vi "CRYSearch for Intersection of Wave.vi"(4 "All points":bool, 6 "Search range":string[](array[string]), 7 "Supress warnings (F)":bool, 9 "Waveform B":T1={"Waveform"={"X0"=0.0, "dX"=0.0, "Y"=[]}, "X data"=1, "Y data"=0, "Y axis"=0, "X unit"="s", "Y unit"="", "Y dB ref"=1.0, "display Y"=TRUE, "display X"=FALSE, "Overload?"=FALSE, "Test Info"="", "Step No."=0, "Name"="", "protected"=FALSE, "Sqc history"=[], "Signal Channel ID"=0, "Plot Settings"={"Color"=0, "Interpolation"=0, "Point Style"=0, "Line Style"=0, "Point Color"=0, "Line Width"=0, "Bar Plot Style"=0, "Fill To"=0}, "AutoProtect"=FALSE} {"Y dB ref" format="%.1f"; "Y axis" items=["Log", "Lin"]; "Y data" items=["dB", "Lin"]; "X data" items=["dB", "Lin"]}, 11 "Waveform A":T1={"Waveform"={"X0"=0.0, "dX"=0.0, "Y"=[]}, "X data"=1, "Y data"=0, "Y axis"=0, "X unit"="s", "Y unit"="", "Y dB ref"=1.0, "display Y"=TRUE, "display X"=FALSE, "Overload?"=FALSE, "Test Info"="", "Step No."=0, "Name"="", "protected"=FALSE, "Sqc history"=[], "Signal Channel ID"=0, "Plot Settings"={"Color"=0, "Interpolation"=0, "Point Style"=0, "Line Style"=0, "Point Color"=0, "Line Width"=0, "Bar Plot Style"=0, "Fill To"=0}, "AutoProtect"=FALSE} {"Y dB ref" format="%.1f"; "Y axis" items=["Log", "Lin"]; "Y data" items=["dB", "Lin"]; "X data" items=["dB", "Lin"]}) -> (3 "Resulting data":T2={"Name"="", "Curve"=[], "X data"=1, "Y data"=1, "Z data"=1, "X axis"=0, "Y axis"=1, "Z axis"=1, "X unit"="Hz", "Y unit"="", "Z unit"="deg.", "X dB ref"=1.0, "Y dB ref"=1.0, "Z dB ref"=1.0, "single val"=FALSE, "protected"=FALSE, "display X"=TRUE, "display Y"=TRUE, "display Z"=TRUE, "Test Info"="", "Step No."=0, "Plot Settings"={"Color"=0, "Interpolation"=0, "Point Style"=0, "Line Style"=0, "Point Color"=0, "Line Width"=0, "Bar Plot Style"=0, "Fill To"=0}, "AutoProtect"=FALSE} {"Z data" items=["dB", "Lin"]; "X data" items=["dB", "Lin"]; "Y data" items=["dB", "Lin"]; "Z dB ref" format="%.1f"; "Z axis" items=["Log", "Lin"]; "X dB ref" format="%.1f"; "X axis" items=["Log", "Lin"]; "Y axis" items=["Log", "Lin"]; "Y dB ref" format="%.1f"; "Curve"."z" format="%.2f"; "Curve"."y" format="%.2f"; "Curve"."x" format="%.2f"})   [LabVIEW 2013]
uses:
  Typedef Control/CRYData Cluster.ctl
  Typedef Control/CRYWaveform Cluster.ctl
  <vilib>/Analysis/7linalg.llb/Solve Linear Equations (single right hand).vi
  <vilib>/Analysis/baseanly.llb/Solve Linear Equations By Cholesky.vi
  <vilib>/Analysis/baseanly.llb/Real Matrix to Compact Array.vi
  <vilib>/Analysis/baseanly.llb/Real Compact Tri-Matrix Linear Eqs.vi
  <vilib>/Analysis/7linalg.llb/Solve Linear Eqs (General).vi
  <vilib>/Analysis/7linalg.llb/Solve Linear Eqs (Gen, single right hand).vi
  <vilib>/Analysis/NI_AALPro.lvlib
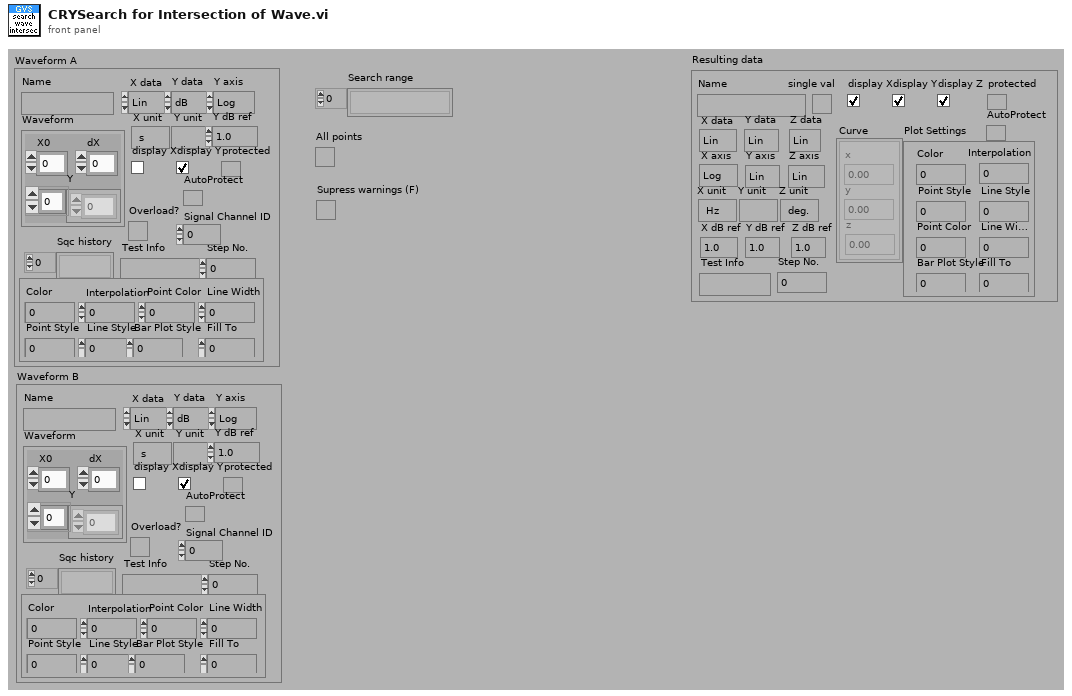
[diagram p1: front panel]
types:
  T1 = typedef "CRYWaveform Cluster.ctl" = cluster{"Waveform":cluster{"X0":dbl, "dX":dbl, "Y":sgl[]}, "X data":u16, "Y data":u16, "Y axis":u16, "X unit":string, "Y unit":string, "Y dB ref":dbl, "display Y":bool, "display X":bool, "Overload?":bool, "Test Info":string, "Step No.":i32, "Name":string, "protected":bool, "Sqc history":string[], "Signal Channel ID":i32, "Plot Settings":cluster{"Color":u32, "Interpolation":u8, "Point Style":u8, "Line Style":u8, "Point Color":u32, "Line Width":u8, "Bar Plot Style":u8, "Fill To":i16}, "AutoProtect":bool}
  T2 = typedef "CRYData Cluster.ctl" = cluster{"Name":string, "Curve":cluster{"x":dbl, "y":dbl, "z":dbl}[], "X data":u16, "Y data":u16, "Z data":u16, "X axis":u16, "Y axis":u16, "Z axis":u16, "X unit":string, "Y unit":string, "Z unit":string, "X dB ref":dbl, "Y dB ref":dbl, "Z dB ref":dbl, "single val":bool, "protected":bool, "display X":bool, "display Y":bool, "display Z":bool, "Test Info":string, "Step No.":i32, "Plot Settings":cluster{"Color":u32, "Interpolation":u8, "Point Style":u8, "Line Style":u8, "Point Color":u32, "Line Width":u8, "Bar Plot Style":u8, "Fill To":i16}, "AutoProtect":bool}
  T3 = enum16{"OK", "Yes", "YesNo", "YesNoCancel", "ReplaceAppend"}
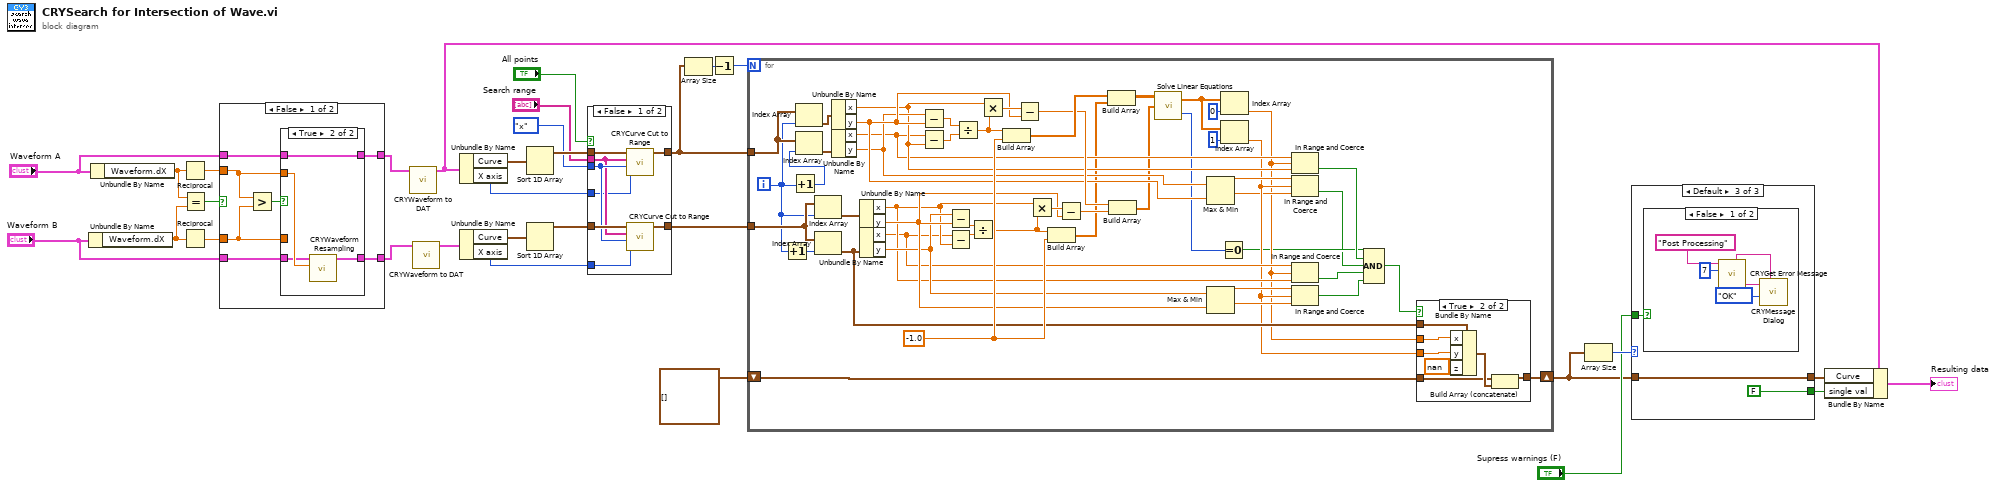
[diagram p0: block diagram]
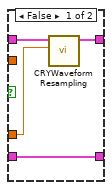
[diagram p3: hidden frame]
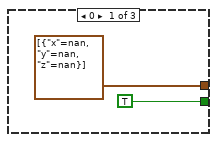
[diagram p5: hidden frame]
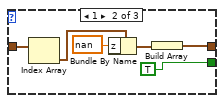
[diagram p6: hidden frame]
diagram:
  n1 = Unbundle By Name("Waveform B") -> ("Waveform.dX"=w13:dbl)
  n2 = Unbundle By Name("Waveform A") -> ("Waveform.dX"=w14:dbl)
  n3 = Reciprocal(x=w14) -> (1/x=w12:dbl)
  n4 = Reciprocal(x=w13) -> (1/x=w11:dbl)
  n5 = Equal?(x=w14, y=w13) -> (x = y?=w1:bool)
  n6 = case shown="False" w1 {
    tunnel: "Waveform A" -> [w38 w48]
    tunnel: "Waveform B" -> [w35 w47]
    tunnel: [w37 w48] -> w10
    tunnel: [w34 w47] -> w9
    tunnel: w12 -> [w36 _]
    tunnel: w11 -> [w33 _]
    frame False {
      n7 = Greater?(x=w36, y=w33) -> (0:w32:bool)
      n8 = case shown="True" w32 {
        tunnel: w38 -> [w42 w46]
        tunnel: [w40 w46] -> w37
        tunnel: w36 -> [_ w45]
        tunnel: w35 -> [w39 w44]
        tunnel: [w39 w43] -> w34
        tunnel: w33 -> [w41 _]
        frame False {
          n9 = call "CRYWaveform Resampling.vi"("New Sampling Rate"=w41, "Wave"=w42) -> ("New Wave"=w40:T1)  [unwired: 9 in]
        }
        frame True {
          n10 = call "CRYWaveform Resampling.vi"("New Sampling Rate"=w45, "Wave"=w44) -> ("New Wave"=w43:T1)  [unwired: 9 in]
        }
      }
    }
    frame True {
    }
  }
  n11 = call "CRYWaveform to DAT.vi"("Waveform In"=w10) -> ("Curve Out"=w8:T2)  [unwired: 10 out]
  n12 = call "CRYWaveform to DAT.vi"("Waveform In"=w9) -> ("Curve Out"=w7:T2)  [unwired: 10 out]
  n13 = Unbundle By Name(w8) -> ("Curve"=w31:cluster{"x":dbl, "y":dbl, "z":dbl}[], "X axis"=w21:u16)
  n14 = Unbundle By Name(w7) -> ("Curve"=w26:cluster{"x":dbl, "y":dbl, "z":dbl}[], "X axis"=w20:u16)
  n15 = Sort 1D Array(array=w31) -> (sorted array=w30:cluster{"x":dbl, "y":dbl, "z":dbl}[])
  n16 = Sort 1D Array(array=w26) -> (sorted array=w25:cluster{"x":dbl, "y":dbl, "z":dbl}[])
  n17 = case shown="False" "All points" {
    tunnel: w30 -> [w56 w58]
    tunnel: [w55 w58] -> w4
    tunnel: enum16{"x", "y", "z"}."x" ("Range variable") -> [w53 _]
    tunnel: "Search range" -> [w52 _]
    tunnel: w25 -> [w54 w57]
    tunnel: [w51 w57] -> w5
    tunnel: w21 -> [w50 _]
    tunnel: w20 -> [w49 _]
    frame False {
      n18 = call "CRYCurve Cut to Range.vi"("Axis type (Lin)"=w50, "Range variable (x)"=w53, "Search range"=w52, "Curve in"=w56) -> ("Cut curve out"=w55:cluster{"x":dbl, "y":dbl, "z":dbl}[])  [unwired: 7 out]
      n19 = call "CRYCurve Cut to Range.vi"("Axis type (Lin)"=w49, "Range variable (x)"=w53, "Search range"=w52, "Curve in"=w54) -> ("Cut curve out"=w51:cluster{"x":dbl, "y":dbl, "z":dbl}[])  [unwired: 7 out]
    }
    frame True {
    }
  }
  n20 = Array Size(array=w4) -> (size(s)=w24:i32)
  n21 = Decrement(x=w24) -> (x-1=w3:i32)
  n22 = for {
    N: w3 -> [_]
    tunnel: w4 -> [w108]
    tunnel: w5 -> [w104]
    shift-right: [w96] -> w2
    shift-left: cluster{"x":dbl, "y":dbl, "z":dbl}[] [] -> [w95]
    i -> [w90]
    w98 = -1.0
    n23 = Increment(x=w90) -> (x+1=w89:i32)
    n24 = Increment(x=w90) -> (x+1=w107:i32)
    n25 = Index Array(array=w108, index=w90) -> (element=w106:cluster{"x":dbl, "y":dbl, "z":dbl})
    n26 = Index Array(array=w108, index=w107) -> (element=w105:cluster{"x":dbl, "y":dbl, "z":dbl})
    n27 = Index Array(array=w104, index=w90) -> (element=w84:cluster{"x":dbl, "y":dbl, "z":dbl})
    n28 = Index Array(array=w104, index=w89) -> (element=w70:cluster{"x":dbl, "y":dbl, "z":dbl})
    n29 = Unbundle By Name(w106) -> ("x"=w92:dbl, "y"=w94:dbl)
    n30 = Unbundle By Name(w105) -> ("x"=w91:dbl, "y"=w93:dbl)
    n31 = Unbundle By Name(w84) -> ("x"=w72:dbl, "y"=w76:dbl)
    n32 = Unbundle By Name(w70) -> ("x"=w71:dbl, "y"=w75:dbl)
    n33 = Subtract(x=w93, y=w94) -> (x-y=w102:dbl)
    n34 = Subtract(x=w91, y=w92) -> (x-y=w103:dbl)
    n35 = Subtract(x=w75, y=w76) -> (x-y=w86:dbl)
    n36 = Subtract(x=w71, y=w72) -> (x-y=w85:dbl)
    n37 = Divide(x=w102, y=w103) -> (x/y=w101:dbl)
    n38 = Divide(x=w86, y=w85) -> (x/y=w87:dbl)
    n39 = Multiply(x=w92, y=w101) -> (x*y=w100:dbl)
    n40 = Build Array(w101, w98) -> (w99:dbl[])
    n41 = Subtract(x=w100, y=w94) -> (x-y=w97:dbl)
    n42 = Multiply(x=w72, y=w87) -> (x*y=w88:dbl)
    n43 = Build Array(w87, w98) -> (w82:dbl[])
    n44 = Subtract(x=w88, y=w76) -> (x-y=w83:dbl)
    n45 = Build Array(w99, w82) -> (w81:dbl[][])
    n46 = Build Array(w97, w83) -> (w80:dbl[])
    n47 = call-poly <vilib>:"Solve Linear Equations.vi"("Known Vector"=w80, "Input Matrix"=w81) -> ("error"=w62:i32, "Solution Vector"=w77:dbl[])  [unwired: 1 in]
    n48 = Max & Min(x=w93, y=w94) -> (max(x,y)=w69:dbl, min(x,y)=w67:dbl)
    n49 = Max & Min(x=w75, y=w76) -> (max(x,y)=w74:dbl, min(x,y)=w73:dbl)
    n50 = Equal To 0?(x=w62) -> (x = 0?=w61:bool)
    n51 = Index Array(array=w77, index=0 ("Index")) -> (element=w66:dbl)
    n52 = Index Array(array=w77, index=1 ("Index")) -> (element=w68:dbl)
    n53 = In Range and Coerce(upper limit=w91, x=w66, lower limit=w92) -> (In Range?=w64:bool)  [unwired: 1 out]
    n54 = In Range and Coerce(upper limit=w69, x=w68, lower limit=w67) -> (In Range?=w59:bool)  [unwired: 1 out]
    n55 = In Range and Coerce(upper limit=w71, x=w66, lower limit=w72) -> (In Range?=w65:bool)  [unwired: 1 out]
    n56 = In Range and Coerce(upper limit=w74, x=w68, lower limit=w73) -> (In Range?=w60:bool)  [unwired: 1 out]
    n57 = Compound Arithmetic op=AND(w61, w64, w59, w65, w60) -> (w63:bool)
    n58 = case shown="True" w63 {
      tunnel: w66 -> [_ w115]
      tunnel: w68 -> [_ w114]
      tunnel: w70 -> [_ w113]
      tunnel: [w109 w111] -> w96
      tunnel: w95 -> [w109 w110]
      frame False {
      }
      frame True {
        n59 = Bundle By Name(cluster=w113, "x"=w115, "y"=w114, "z"=nan) -> (w112:cluster{"x":dbl, "y":dbl, "z":dbl})
        n60 = Build Array (concatenate)(w110, w112) -> (w111:cluster{"x":dbl, "y":dbl, "z":dbl}[])
      }
    }
  }
  n61 = Array Size(array=w2) -> (size(s)=w23:i32)
  n62 = case shown="Default" w23 {
    tunnel: w2 -> [_ w124 w125]
    tunnel: [cluster{"x":dbl, "y":dbl, "z":dbl}[] [{"x"=nan, "y"=nan, "z"=nan}] w119 w125] -> w22
    tunnel: "Supress warnings (F)" -> [_ _ w127]
    tunnel: [TRUE ("Bundle Element") TRUE ("Bundle Element") FALSE ("Bundle Element")] -> w19
    frame 0 {
    }
    frame 1 {
      n63 = Index Array(array=w124) -> (element=w123:cluster{"x":dbl, "y":dbl, "z":dbl})  [unwired: 1 in]
      n64 = Bundle By Name(cluster=w123, "z"=nan) -> (w121:cluster{"x":dbl, "y":dbl, "z":dbl})
      n65 = Build Array(w121) -> (w119:cluster{"x":dbl, "y":dbl, "z":dbl}[])
    }
    frame Default {
      n66 = case shown="False" w127 {
        frame False {
          n67 = call "CRYGet Error Message.vi"("Error No"=7, "Kind"="Post Processing") -> ("Message Sub 3"=w130:string, "Window Title"=w128:string)  [unwired: 4 in, 4 out]
          n68 = call "CRYMessage Dialog.vi"("Window Title"=w128, "YesNoCancel"=T3."OK", "Message Content"=w130) -> ()  [unwired: 7 in, 2 out]
        }
        frame True {
        }
      }
    }
  }
  n69 = Bundle By Name(cluster=w8, "Curve"=w22, "single val"=w19) -> (→"Resulting data":T2)
